vi "motor safety.vi"(0 "Desired Rate":dbl, 1 "Forward Limit":dbl, 2 "Reverse Limit":dbl, 3 "Cutoff Rate":dbl=0.2, 4 "Max Rate":dbl=50.0, 5 "Min Rate":dbl, 6 "Encoder Refnum":string) -> (7 "Encoder Disconnected":bool, 9 "No Rate Read":bool, 11 "At Distance Limit":bool, 13 "Encoder Directional Issue":bool, 14 "Rate Output":dbl, 19 "Input Out of Range":bool)   [LabVIEW 2014]
doc: "This VI provides two types of safety for your motors. An encoder for the motor is required. If the encoder reference is innalid, the motor won't be allowed to run. \nThe first safetyis a distance limit. The forward and reverse limit parameters specify the max and min valus for the encoder distance to read until the motor is stopped and only allowed to move away from its limit. \nThe second safety is an encoder safety. The Cutoff Rate parameter is the maximum value allowed to be sent to the motor without a response seen from the encoder. So, if the code is trying to set a value higher than this parameter and the encoder doesn't register a response, the motor will be disabled. It will be reenabled when movement is registered from the encoder. This safety will also permanately disable the motor if the encoder reads some inanely high rate. Consider a replacement...."
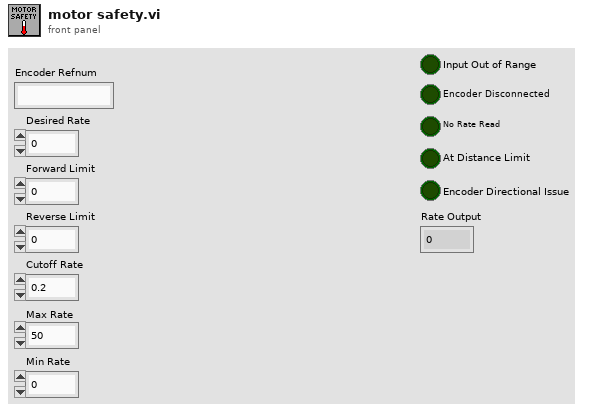
[diagram p1: front panel]
types:
  T1 = typedef "WPI_EncoderDevRef.ctl" = cluster{"DevStatus":errorcluster, "EncoderIndex":T2, "CounterIndex":T3, "DistancePerCount":dbl, "Decoding Type":T4}
  T2 = typedef "FPGA_EncoderIdx.ctl" = enum8{"Enc 0", "Enc 1", "Enc 2", "Enc 3", "Enc 4", "Enc 5", "Enc 6", "Enc 7", "Invalid"}
  T3 = typedef "FPGA_CounterCtrSystemIndex.ctl" = enum8{"Ctr 0", "Ctr 1", "Ctr 2", "Ctr 3", "Ctr 4", "Ctr 5", "Ctr 6", "Ctr 7", "Invalid"}
  T4 = typedef "WPI_EncoderType.ctl" = enum16{"1x", "2x", "4x"}
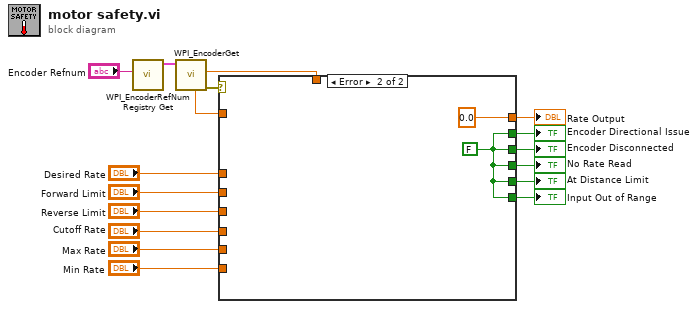
[diagram p0: block diagram]
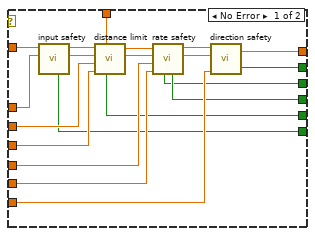
[diagram p2: hidden frame]
diagram:
  n1 = call <vilib>:"WPI_EncoderRefNum Registry Get.vi"("refnum name"="Encoder Refnum") -> ("EncoderDevRef"=w16:T1)  [unwired: 9 in, 1 out]
  n2 = call <vilib>:"WPI_EncoderGet.vi"("EncoderDevRef"=w16) -> ("error out"=w8:errorcluster, "Distance"=w13:dbl, "Rate"=w15:dbl)  [unwired: 5 in, 3 out]
  n3 = case shown="Error" w8 {
    tunnel: w15 -> [w26 _]
    tunnel: "Desired Rate" -> [w22 _]
    tunnel: w13 -> [w35 _]
    tunnel: [w32 0.0 ("Output Rate")] -> w12
    tunnel: "Forward Limit" -> [w23 _]
    tunnel: "Reverse Limit" -> [w24 _]
    tunnel: "Cutoff Rate" -> [w31 _]
    tunnel: [w19 w38] -> w7
    tunnel: [w20 w38] -> w6
    tunnel: "Max Rate" -> [w29 _]
    tunnel: "Min Rate" -> [w28 _]
    tunnel: [w37 w38] -> w3
    tunnel: [w21 w38] -> w2
    tunnel: [w18 w38] -> w1
    frame No Error {
      n4 = call "input safety.vi"("Desired Rate"=w22, "Encoder Rate"=w26) -> ("Safe Rate"=w25:dbl, "Encoder Rate Out"=w27:dbl, "Input Out of Range"=w18:bool)  [unwired: 7 in]
      n5 = call "distance limit.vi"("Encoder Rate"=w27, "Encoder Distance"=w35, "Desired Rate"=w25, "Forward Limit"=w23, "Reverse Limit"=w24) -> ("At Distance Limit"=w21:bool, "Encoder Rate Out"=w36:dbl, "Output Rate"=w30:dbl)  [unwired: 1 in]
      n6 = call "rate safety.vi"("Max Rate"=w29, "Cutoff Rate"=w31, "Desired Rate"=w30, "Encoder Rate"=w36) -> ("Output Rate"=w33:dbl, "Encoder Rate Out"=w34:dbl, "No Rate Read"=w20:bool, "Encoder Failure"=w19:bool)  [unwired: 4 in]
      n7 = call "direction safety.vi"("Min Rate"=w28, "Desired Rate"=w33, "Encoder Rate"=w34) -> ("Encoder Directional Issue"=w37:bool, "Super Safe Rate"=w32:dbl)  [unwired: 1 in]
    }
    frame Error {
      w38 = FALSE ("Cutoff Tripped")
    }
  }
  "Rate Output" <- w12
  "Encoder Disconnected" <- w7
  "No Rate Read" <- w6
  "Encoder Directional Issue" <- w3
  "At Distance Limit" <- w2
  "Input Out of Range" <- w1
